vi "mul.vi"() -> ()   [LabVIEW 2026]
panel:
  out "output":dbl
  in  "b":dbl
  in  "a":dbl
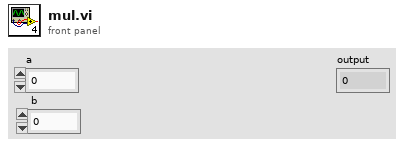
[diagram p1: front panel]
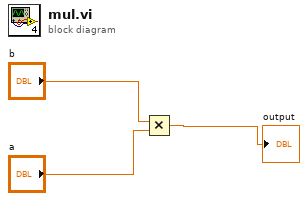
[diagram p0: block diagram]
diagram:
  n1 = Multiply(x="b", y="a") -> (x*y=→"output":dbl)
